vi "WriteDO.vi"(8 "error in (no error)":errorcluster, 9 "DO Value (True)":bool=TRUE, 10 "Output":T1, 11 "VISA resource name":refnum<visa-resource-name>) -> (0 "error out":errorcluster, 3 "VISA resource name out":refnum<visa-resource-name>)   [LabVIEW 2020, in "HandsOnPi2040.lvlib"]
doc: "Establishes communication with the instrument and optionally performs an instrument identification query and/or an instrument reset. It also places the instrument in a default state needed for other instrument driver operations. Therefore, call this VI before calling other instrument driver VIs for this instrument. Generally, you need to call the <b>Initialize</b> VI only once at the beginning of an application."
uses:
  <instrlib>/HandsOnPi2040/HandsOnPi2040.lvlib
  <instrlib>/HandsOnPi2040/Public/DigOuts.ctl
panel:
  # "Input"
  # "Output"
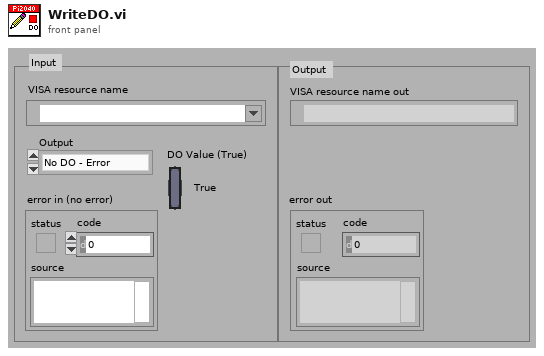
[diagram p1: front panel]
types:
  T1 = typedef "HandsOnPi2040.lvlib/DigOuts.ctl" = enum16{"No DO - Error", "DO1", "DO2", "DO3", "DO4", "BEEP"}
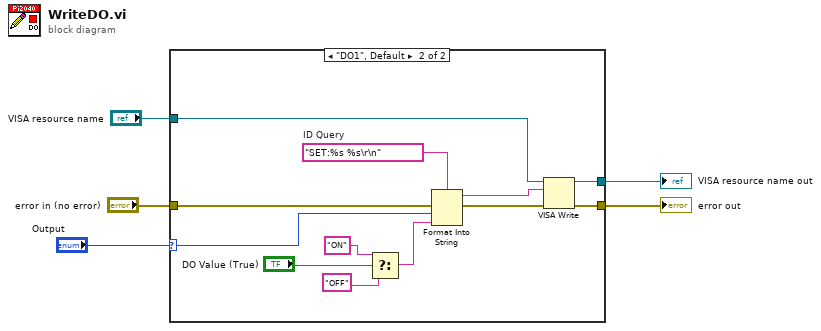
[diagram p0: block diagram]
diagram:
  n1 = case shown="\"DO1\", Default" "Output" {
    selector: "Output" -> [_ w19]
    tunnel: [w7 w12] -> w2
    tunnel: [w6 w11] -> w3
    tunnel: "VISA resource name" -> [w6 w10]
    tunnel: "error in (no error)" -> [w7 w9]
    frame "No DO - Error" {
    }
    frame "DO1", Default {
      w18 = "SET:%s %s\r\n"  # ID Query
      n2 = Select(t="ON", s="DO Value (True)", f="OFF") -> (s? t:f=w14:string)
      n3 = Format Into String(format string=w18, error in=w9, w19, w14) -> (resulting string=w8:string, error out=w13:errorcluster)  [unwired: 1 in]
      n4 = VISA Write(VISA resource name=w10, write buffer=w8, error in (no error)=w13) -> (VISA resource name out=w11:refnum<visa-resource-name>, error out=w12:errorcluster)  [unwired: 1 out]
    }
  }
  "VISA resource name out" <- w3
  "error out" <- w2
